vi "Get All Latest Values.vi"(0 "reference in":refnum<class "Reporter.lvclass">, 5 "error in (no error)":errorcluster) -> (14 "reference out":refnum<class "Reporter.lvclass">, 16 "All Latest Values":dbl[](array[numeric]), 19 "error out":errorcluster)   [LabVIEW 2018, in "Reporter.lvclass"]
uses:
  Reporter.lvclass
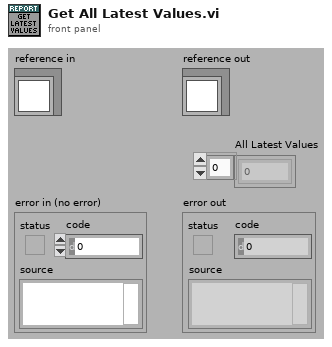
[diagram p1: front panel]
types:
  T1 = typedef "Reporter.lvclass/ObjectAttributes.ctl" = cluster{"LCR":refnum<class "BKP-891 LCR Meter.lvclass">, "PSU":refnum<class "BKP-911x Power Supply.lvclass">, "NI-DAQmx":refnum<class "NI-DAQmx.lvclass">, "Signal List":T2[], "Latest Values":dbl[], "All Latest Values":dbl[], "All Signal List":T2[], "Report Directory":path, "Report File Ref":refnum<file>}
  T2 = typedef "IO Signal List.ctl" = enum16{"Timestamp", "PSU_FB_U_VDC", "PSU_FB_I_AMP", "PSU_FB_W_WATT", "PSU_CMD_U_VDC", "PSU_CMD_I_AMP", "PSU_CMD_OUTPUT", "LCR_PRIMARY", "LCR_SECONDARY", "UV_R_Ohm", "UW_R_Ohm", "VW_R_Ohm", "UV_L_H", "UW_L_H", "VW_L_H", "U_U_VDC", "V_U_VDC", "W_U_VDC", "U_I_AMP", "V_I_AMP", "W_I_AMP", "PWM_CMD_DC_%", "PWM_CMD_VDC", "PWM_CMD_Hz", "PWM_FB_DC_%", "PWM_FB_VDC", "PWM_FB_Hz", "DO_RELAY_U_LCR_A", "DO_RELAY_V_LCR_A", "DO_RELAY_V_LCR_B", "DO_RELAY_W_LCR_B", "DIFF_UV_UW_L_H", "DIFF_UV_VW_L_H", "DIFF_UW_VW_L_H", "DIFF_UV_UW_R_Ohm", "DIFF_UV_VW_R_Ohm", "DIFF_UW_VW_R_Ohm", "DIFF_UV_U_VDC", "DIFF_UW_U_VDC", "DIFF_VW_U_VDC"}
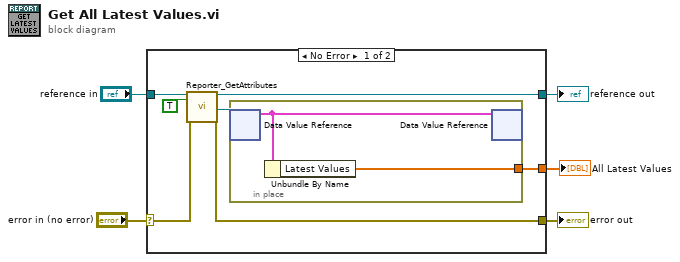
[diagram p0: block diagram]
diagram:
  n1 = case shown="No Error" "error in (no error)" {
    selector: "error in (no error)" -> [w12 w16]
    tunnel: [w11 w16] -> w4
    tunnel: [w9 w15] -> w2
    tunnel: "reference in" -> [w10 w15]
    tunnel: [w6 _] -> w1
    frame No Error {
      n2 = call "Reporter_GetAttributes.vi"("reference in"=w10, "OnlyGetDvrReference(False)"=TRUE, "error in (no error)"=w12) -> ("reference out"=w9:refnum<class "Reporter.lvclass">, "DataRef"=w8:refnum<data-value>, "error out"=w11:errorcluster)  [unwired: 13 in, 1 out]
      n3 = in-place {
        in-place-border: [w14] -> w6
        n4 = in-place-dvr #1(w8) -> (w13:T1)  [unwired: 1 out]
        n5 = Unbundle By Name(w13) -> ("Latest Values"=w14:dbl[])
        n6 = in-place-dvr #1(w13) -> ()  [unwired: 2 out]
      }
    }
    frame Error {
    }
  }
  "error out" <- w4
  "reference out" <- w2
  "All Latest Values" <- w1
